vi "Connect.vi"(8 "error in":errorcluster) -> (0 "error out":errorcluster, 3 "Data Cluster":T1)   [LabVIEW 2017, in "Akwizycja.lvlib"]
uses:
  Akwizycja.lvlib
  <vilib>/Plasmionique/MB Master/MB_Master_Serial/MB_Master_Serial.lvclass
  <vilib>/Utility/config.llb/NI_LVConfig.lvlib
panel:
  in  "Fuel Flow":dbl[][][](array[numeric])
  in  "Init array":refnum<class "MB_Master_Serial.lvclass">[](array[class])
  in  "Array of temperatures":dbl[][][](array[numeric])
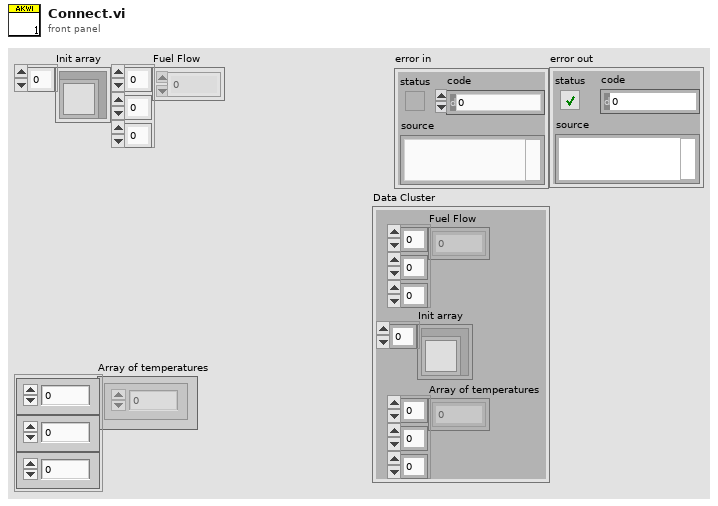
[diagram p1: front panel]
types:
  T1 = cluster{"Fuel Flow":dbl[][][], "Init array":refnum<class "MB_Master_Serial.lvclass">[], "Array of temperatures":dbl[][][]}
  T2 = typedef "NI_LVConfig.lvlib/Config Data RefNum.ctl" = refnum<k1>
  T3 = cluster{"baud rate (bps)":u32, "stop bits":u16, "parity":u16, "flow control":u16, "timeout":u32, "retries":i32}
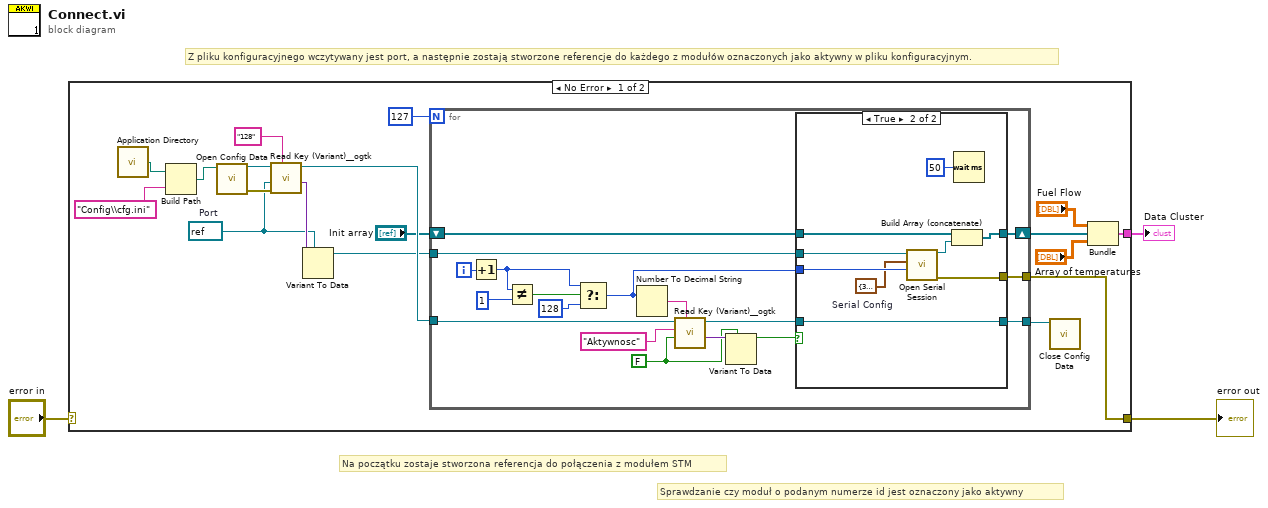
[diagram p0: block diagram]
diagram:
  # "Na początku zostaje stworzona referencja do połączenia z modułem STM"
  # "Sprawdzanie czy moduł o podanym numerze id jest oznaczony jako aktywny"
  # "Z pliku konfiguracyjnego wczytywany jest port, a następnie zostają stworzone referencje do każdego z modułów oznaczonych jako aktywny w pliku konfiguracyjnym."
  n1 = case shown="No Error" "error in" {
    selector: "error in" -> [_ w51]
    tunnel: [w19 _] -> w1
    tunnel: [w17 w51] -> w2
    frame No Error {
      w6 = refnum<visa-resource-name> refnum  # Port
      n2 = call <vilib>:"Application Directory.vi"() -> ("Application Directory"=w16:path)
      n3 = Build Path(base path=w16, name or relative path="Config\\cfg.ini") -> (appended path=w14:path)
      n4 = call <vilib>:"Open Config Data.vi"("configuration file path"=w14) -> ("error out"=w12:errorcluster, "refnum"=w13:T2)  [unwired: 8 in, 1 out]
      n5 = call <userlib>:"Read Key (Variant)__ogtk.vi"("section"="128", "error in (no error)"=w12, "type"=w6, "refnum"=w13) -> ("key-value"=w10:variant, "refnum out"=w21:T2)  [unwired: 4 in, 2 out]
      n6 = Variant To Data(type=w6, Variant=w10) -> (data=w9:refnum<visa-resource-name>)  [unwired: 1 in, 1 out]
      n7 = for {
        N: 127 -> [_]
        tunnel: w9 -> [w28]
        shift-right: [w37] -> w20
        shift-left: "Init array" -> [w38]
        tunnel: [w39] -> w17
        tunnel: w21 -> [w36]
        tunnel: [w30] -> w5
        i -> [w27]
        w29 = FALSE
        n8 = Increment(x=w27) -> (x+1=w25:i32)
        n9 = Not Equal?(x=w25, y=1) -> (x != y?=w23:bool)
        n10 = Select(t=w25, s=w23, f=128) -> (s? t:f=w26:i32)
        n11 = Number To Decimal String(number=w26) -> (decimal integer string=w34:string)  [unwired: 1 in]
        n12 = call <userlib>:"Read Key (Variant)__ogtk.vi"("section"=w34, "type"=w29, "key (optional)"="Aktywnosc", "refnum"=w36) -> ("key-value"=w33:variant, "refnum out"=w31:T2)  [unwired: 4 in, 2 out]
        n13 = Variant To Data(type=w29, Variant=w33) -> (data=w32:bool)  [unwired: 1 in, 1 out]
        n14 = case shown="True" w32 {
          tunnel: w28 -> [_ w49]
          tunnel: [_ w48] -> w39
          tunnel: w38 -> [w41 w47]
          tunnel: [w41 w45] -> w37
          tunnel: w26 -> [_ w50]
          tunnel: w31 -> [w40 w43]
          tunnel: [w40 w43] -> w30
          frame False {
          }
          frame True {
            w44 = T3 {"baud rate (bps)"=38400, "stop bits"=10, "parity"=0, "flow control"=0, "timeout"=1000, "retries"=1}  # Serial Config
            n15 = call <vilib>:"Open Serial Session.vi"("Slave ID"=w50, "Serial Config"=w44, "VISA Resource"=w49) -> ("Error out"=w48:errorcluster, "MB_Serial session"=w46:refnum<class "MB_Master_Serial.lvclass">)  [unwired: 7 in]
            n16 = Build Array (concatenate)(w47, w46) -> (w45:refnum<class "MB_Master_Serial.lvclass">[])
            n17 = Wait (ms)(milliseconds to wait=u32 50) -> ()  [unwired: 1 out]
          }
        }
      }
      n18 = call <vilib>:"Close Config Data.vi"("refnum"=w5) -> ()  [unwired: 9 in, 2 out]
      n19 = Bundle("Fuel Flow"="Fuel Flow", "Init array"=w20, "Array of temperatures"="Array of temperatures") -> (w19:T1)  [unwired: 1 in]
    }
    frame Error {
    }
  }
  "error out" <- w2
  "Data Cluster" <- w1
